vi "全局 水样时间.vi"() -> ()   [LabVIEW 2016, in "数据传输系统-06.lvlib"]
panel:
  in  "ADCP流程":string
  out "循环运行次数":i32
  in  "上传动作":string
  in  "ADCP数据时间":string
  in  "在线ADCP分层数据时间":string
  in  "海流计流程":string
  in  "一体式气象时间":string
  in  "波浪仪数据时间":string
  out "队列数量":u32
  out "元素":string[](array[string])
  in  "N个五分钟":u32
  in  "海流计数据时间":string
  in  "仪器":string
  in  "数据查询指令":string
  in  "数据查表起始时间":T1
  in  "剖面数据时间":string
  in  "剖面多参数数据时间":string
  in  "水样数据索引":T2
  in  "选择发送的参数":string
  in  "小时数据时间":string
  in  "时间":string
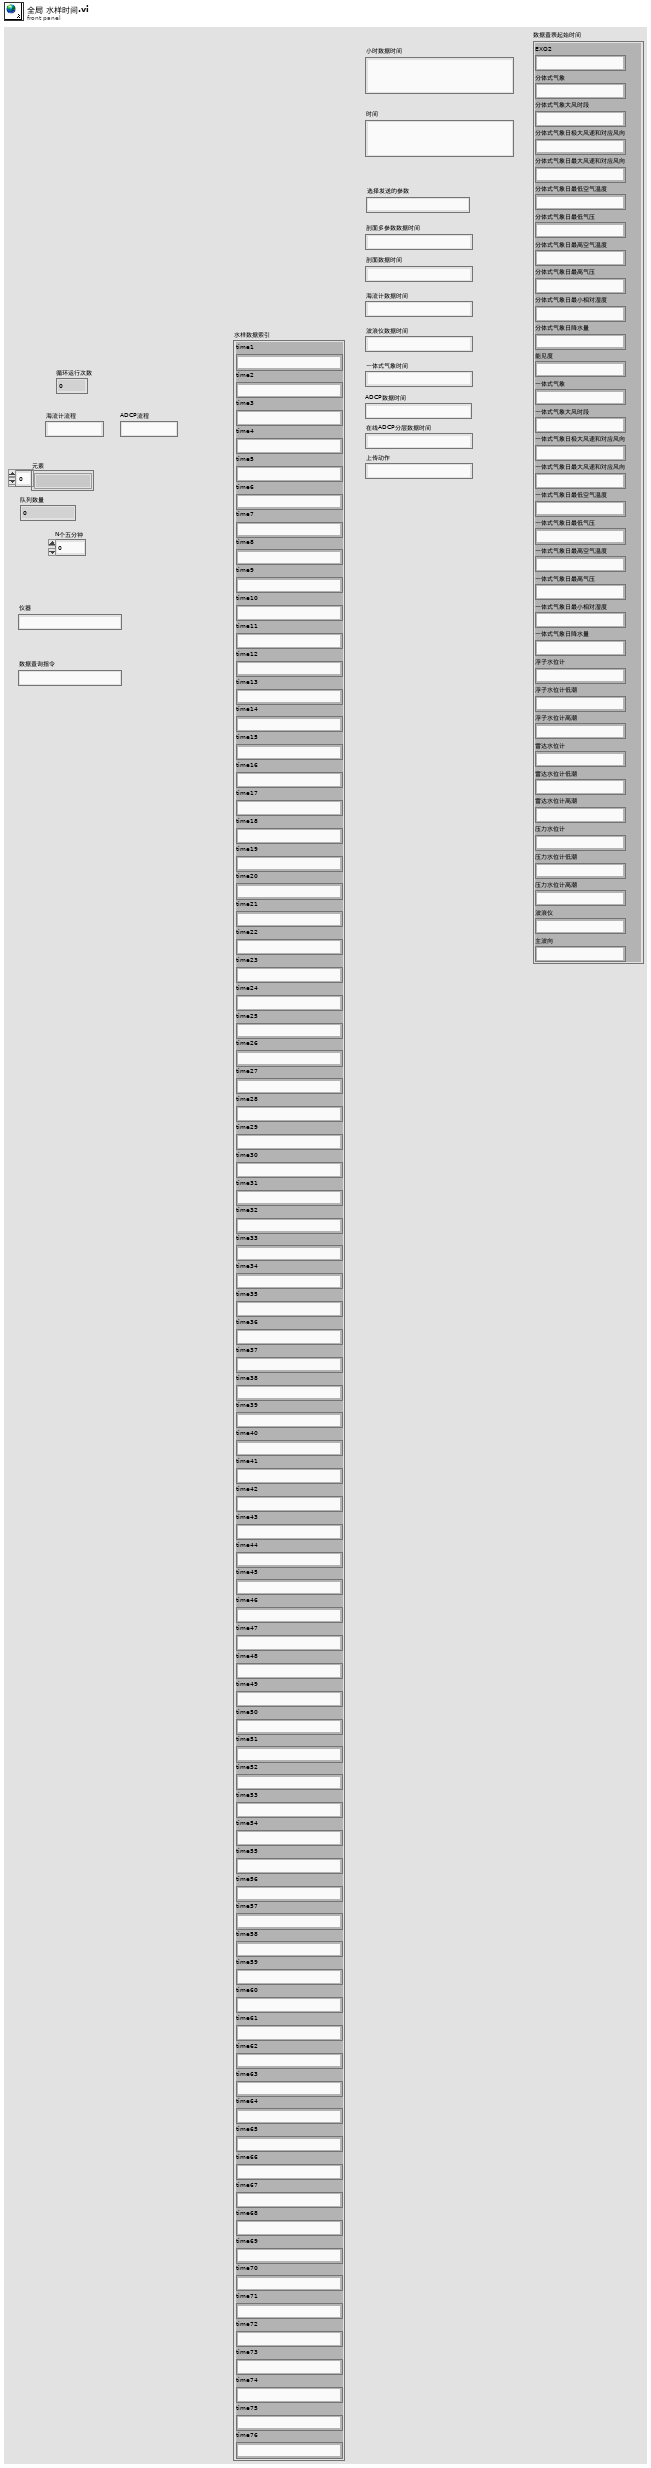
[diagram p1: front panel]
types:
  T1 = cluster{"EXO2":string, "分体式气象":string, "分体式气象大风时段":string, "分体式气象日极大风速和对应风向":string, "分体式气象日最大风速和对应风向":string, "分体式气象日最低空气温度":string, "分体式气象日最低气压":string, "分体式气象日最高空气温度":string, "分体式气象日最高气压":string, "分体式气象日最小相对湿度":string, "分体式气象日降水量":string, "能见度":string, "一体式气象":string, "一体式气象大风时段":string, "一体式气象日极大风速和对应风向":string, "一体式气象日最大风速和对应风向":string, "一体式气象日最低空气温度":string, "一体式气象日最低气压":string, "一体式气象日最高空气温度":string, "一体式气象日最高气压":string, "一体式气象日最小相对湿度":string, "一体式气象日降水量":string, "浮子水位计":string, "浮子水位计低潮":string, "浮子水位计高潮":string, "雷达水位计":string, "雷达水位计低潮":string, "雷达水位计高潮":string, "压力水位计":string, "压力水位计低潮":string, "压力水位计高潮":string, "波浪仪":string, "主波向":string}
  T2 = cluster{"time1":string, "time2":string, "time3":string, "time4":string, "time5":string, "time6":string, "time7":string, "time8":string, "time9":string, "time10":string, "time11":string, "time12":string, "time13":string, "time14":string, "time15":string, "time16":string, "time17":string, "time18":string, "time19":string, "time20":string, "time21":string, "time22":string, "time23":string, "time24":string, "time25":string, "time26":string, "time27":string, "time28":string, "time29":string, "time30":string, "time31":string, "time32":string, "time33":string, "time34":string, "time35":string, "time36":string, "time37":string, "time38":string, "time39":string, "time40":string, "time41":string, "time42":string, "time43":string, "time44":string, "time45":string, "time46":string, "time47":string, "time48":string, "time49":string, "time50":string, "time51":string, "time52":string, "time53":string, "time54":string, "time55":string, "time56":string, "time57":string, "time58":string, "time59":string, "time60":string, "time61":string, "time62":string, "time63":string, "time64":string, "time65":string, "time66":string, "time67":string, "time68":string, "time69":string, "time70":string, "time71":string, "time72":string, "time73":string, "time74":string, "time75":string, "time76":string}
diagram:
